vi "WriteServoAngle.vi"() -> ()   [LabVIEW 2012]
uses:
  <vilib>/FPGAPlugInAG/sbRIO-9642/niLvFpga_Open_sbRIO-9642.vi
  <vilib>/rvi/interface/common/dynamic/niFpgaDynamicAddResources.vi
  <vilib>/Utility/error.llb/Error Cluster From Error Code.vi
  <vilib>/rvi/errors/niLvFpgaAdjustHostInterfaceError.vi
  <vilib>/rvi/interface/nirviOpenFPGA/nirviOpenFPGA.xnode
  FPGA Bitfiles/NatesProject1_FPGATarget_FPGAConfig_9WlgTycNURQ.lvbitx
  FPGA Config.vi
  <vilib>/rvi/interface/nirviReadWriteControl/nirviReadWriteControl.xnode
  NiFpgaLv.dll
  <vilib>/rvi/interface/Simulation/niFpgaSimulationCallBeginRW.vi
panel:
  out "Numeric":i32
  in  "Angle In(Deg)":dbl(slide) scale=-90.0..90.0
  in  "stop":bool
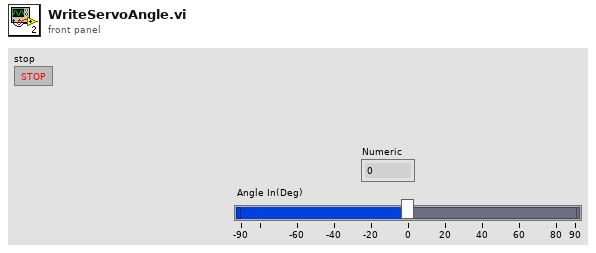
[diagram p1: front panel]
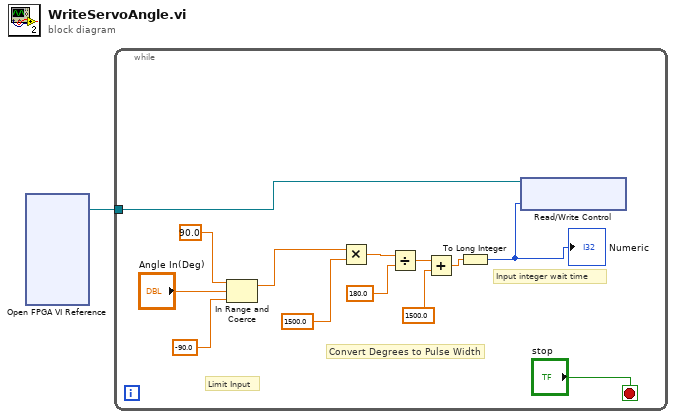
[diagram p0: block diagram]
diagram:
  n1 = xnode "Open FPGA VI Reference"() -> ("FPGA VI Reference Out"=w1:refnum<k20>)  [unwired: 2 in, 1 out]
  n2 = while {
    tunnel: w1 -> [w13]
    stop <- "stop" stop-if-true
    # "Input integer wait time"
    # "Convert Degrees to Pulse Width"
    # "Limit Input"
    n3 = In Range and Coerce(upper limit=90.0, x="Angle In(Deg)", lower limit=-90.0) -> (coerced(x)=w11:dbl)  [unwired: 1 out]
    n4 = Multiply(x=w11, y=1500.0) -> (x*y=w8:dbl)
    n5 = Divide(x=w8, y=180.0) -> (x/y=w4:dbl)
    n6 = Add(x=w4, y=1500.0) -> (x+y=w3:dbl)
    n7 = To Long Integer(number=w3) -> (32bit integer=w5:i32)
    "Numeric" <- w5
    n8 = xnode "Read/Write Control"("FPGA VI Reference In"=w13, "Pulse Width(uSec)"=w5) -> ()  [unwired: 1 in, 2 out]
  }
